vi "Write String.vi"(8 "error in (no error)":errorcluster, 10 "Input":string, 11 "JSON Lexer in":refnum<class "JSON Lexer.lvclass">) -> (0 "error out":errorcluster, 3 "JSON Lexer out":refnum<class "JSON Lexer.lvclass">)   [LabVIEW 2019, in "JKI JSON Serialization.lvlib" / "JSON Lexer.lvclass"]
doc: "JKI JSON 1.1.10.37\nTomi Maila - JKI\nCopyright (c) 2017, JKI"
uses:
  JSON Lexer.lvclass
  JSON Token.ctl
  JSON Token Type.ctl
  Unicode/UTF-8 String/UTF-8 String.lvclass/UTF-8 String.ctl
  JSON Lexer.lvclass/JSON Lexer.ctl
  Unicode/UTF-8 String/UTF-8 String.lvclass
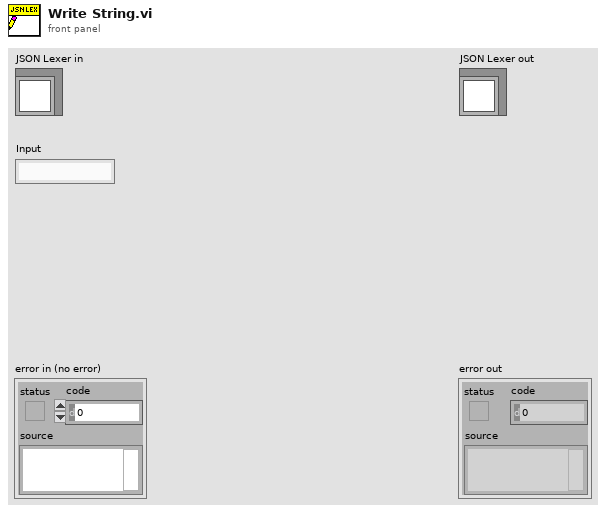
[diagram p1: front panel]
types:
  T1 = typedef "JKI JSON Serialization.lvlib/JSON Lexer.lvclass/JSON Token.ctl" = cluster{"Token Type":T2, "Token Value":string}
  T2 = typedef "JKI JSON Serialization.lvlib/JSON Lexer.lvclass/JSON Token Type.ctl" = enum32{"unknown", "comma", "end-label", "begin-object", "end-object", "begin-array", "end-array", "quoted-string", "boolean", "exponential-number", "decimal-number", "integer-number", "special-number", "null", "symbol", "whitespace", "EOF"}
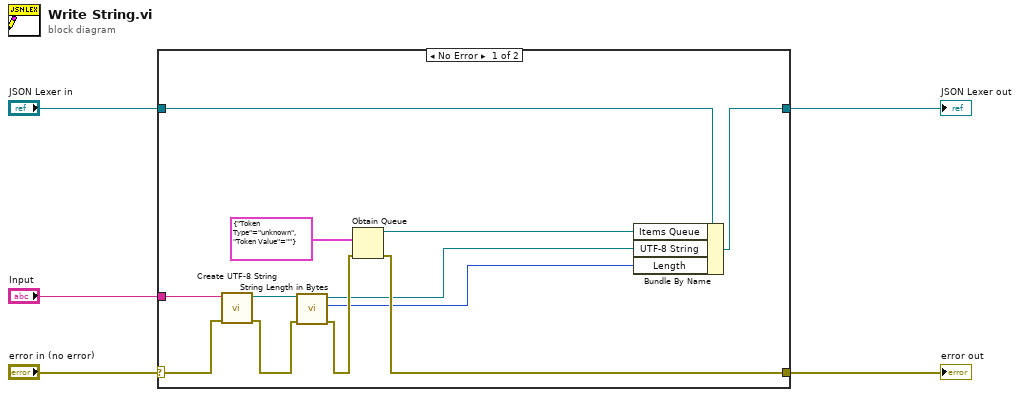
[diagram p0: block diagram]
diagram:
  n1 = case shown="No Error" "error in (no error)" {
    selector: "error in (no error)" -> [w11 w19]
    tunnel: [w16 w19] -> w2
    tunnel: [w14 w18] -> w1
    tunnel: "JSON Lexer in" -> [w15 w18]
    tunnel: "Input" -> [w12 _]
    frame No Error {
      n2 = call "Create UTF-8 String.vi"("error in (no error)"=w11, "UTF-8 String"=w12) -> ("error out"=w9:errorcluster, "UTF-8 String"=w10:refnum<class "UTF-8 String.lvclass">)  [unwired: 8 in]
      n3 = call "String Length in Bytes.vi"("error in (no error)"=w9, "UTF8 in"=w10) -> ("error out"=w8:errorcluster, "Length in Bytes"=w6:i32, "UTF8 out"=w7:refnum<class "UTF-8 String.lvclass">)  [unwired: 7 in]
      n4 = Obtain Queue(element data type=T1 {"Token Type"=enum."unknown", "Token Value"=""} ("Item"), error in (no error)=w8) -> (queue out=w13:refnum<queue>, error out=w16:errorcluster)  [unwired: 3 in, 1 out]
      n5 = Bundle By Name(cluster=w15, "Items Queue"=w13, "UTF-8 String"=w7, "Length"=w6) -> (w14:refnum<class "JSON Lexer.lvclass">)
    }
    frame Error {
    }
  }
  "error out" <- w2
  "JSON Lexer out" <- w1
